vi "FPGA_target_set_stop_output.vi"(9 "connector0_data":T1, 11 "connector1_data":T1) -> ()   [LabVIEW 2014]
doc: "writes the pattern data to the outputs in case the pattern output is stopped"
uses:
  FPGA_32BitPattern_data_type.ctl
  <vilib>/rvi/eio/common/nirviEmuTemplateMethod_errors.vi
  <vilib>/eio/EIONode/EIONode.xnode
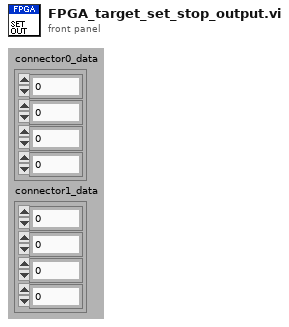
[diagram p1: front panel]
types:
  T1 = typedef "FPGA_32BitPattern_data_type.ctl" = cluster{"port0":u8, "port1":u8, "port2":u8, "port3":u8}
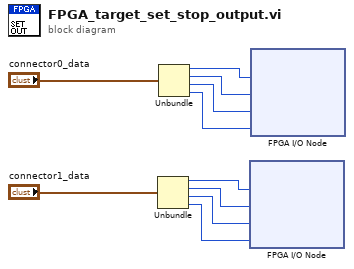
[diagram p0: block diagram]
diagram:
  n1 = Unbundle("connector1_data") -> ("port0"=w1:u8, "port1"=w2:u8, "port2"=w3:u8, "port3"=w4:u8)
  n2 = Unbundle("connector0_data") -> ("port0"=w8:u8, "port1"=w7:u8, "port2"=w6:u8, "port3"=w5:u8)
  n3 = xnode ("FPGA I/O Node")("DO_56-63"=w1, "DO_48-55"=w2, "DO_40-47"=w3, "DO_32-39"=w4) -> ()  [unwired: 4 in, 4 out]
  n4 = xnode ("FPGA I/O Node")("DO_24-31"=w8, "DO_16-23"=w7, "DO_08-15"=w6, "DO_00-07"=w5) -> ()  [unwired: 4 in, 4 out]
